vi "CreatePublicEvents.vi"(8 "error in (no error)":errorcluster, 11 "Generator":refnum<class "Generator.lvclass">) -> (0 "error out":errorcluster, 3 "Generator out":refnum<class "Generator.lvclass">)   [LabVIEW 2019, in "Generator.lvclass"]
uses:
  Generator.lvclass
  typedefs/AO.Channel--Cluster--Array.ctl
  typedefs/AO.Channel--Cluster.ctl
  typedefs/AO.Channel.Function--Enum.ctl
  typedefs/Waveforms--Cluster.ctl
  Generator.lvclass/Generator.ctl
  <vilib>/JKI/JKI SMO/SMO/SMO.lvclass
  typedefs/Generator.Sweep Status--enum.ctl
panel:
  # "For instructions on how to use the JKI State Machine Objects, examples and video tutorials, visit:\nhttp://jki.net/state-machine-objects/\n\nJKI State Machine Objects™\nhttp://jki.net/state-machine-objects/\nCopyright (C) 2005-2015, JKI <info@jki.net>\nALL RIGHTS RESERVED"
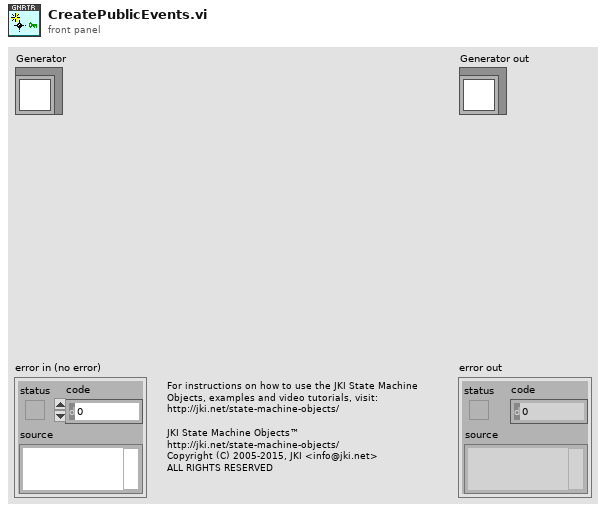
[diagram p1: front panel]
types:
  T1 = typedef "Generator.lvclass/Generator.Sweep Status--enum.ctl" = enum16{"idle", "initializing", "waiting", "sweeping", "stopping"}
  T2 = typedef "Generator.lvclass/Waveforms--Cluster.ctl" = cluster{"AO":waveform(dbl)[], "REF_X":waveform(dbl)[], "REF_Y":waveform(dbl)[]}
  T3 = typedef "Generator.lvclass/AO.Channel--Cluster--Array.ctl" = T4[]
  T4 = typedef "Generator.lvclass/AO.Channel--Cluster.ctl" = cluster{"Enable?":bool, "Channel":i32, "Amplitude":dbl, "Offset":dbl, "Frequency":dbl, "Phase":dbl, "Function":T5, "Sweeping?":bool, "Limit AC?":bool, "Limit DC?":bool, "Duty Cycle?":bool, "Duty Cycle":dbl}
  T5 = typedef "Generator.lvclass/AO.Channel.Function--Enum.ctl" = enum16{"sine", "square", "triangle", "saw"}
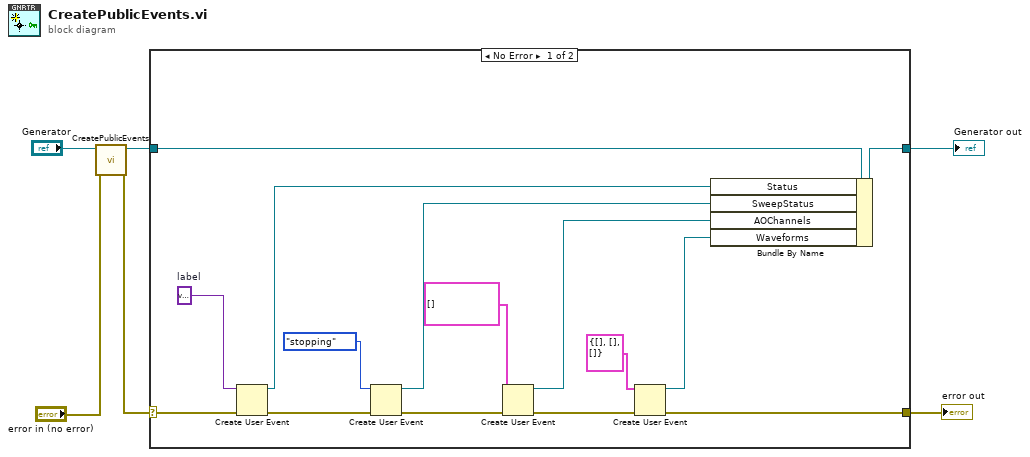
[diagram p0: block diagram]
diagram:
  n1 = call-parent "CreatePublicEvents.vi"("error in (no error)"="error in (no error)", "SMO"="Generator") -> ("error out"=w1:errorcluster, "SMO out"=w5:refnum<class "Generator.lvclass">)  [unwired: 8 in]
  n2 = case shown="No Error" w1 {
    selector: w1 -> [w20 w23]
    tunnel: [w12 w23] -> w3
    tunnel: [w21 w22] -> w4
    tunnel: w5 -> [w18 w22]
    frame No Error {
      w17 = variant  # label
      n3 = Create User Event(user event datatype=w17, error in=w20) -> (user event=w19:refnum<user-event>, error out=w16:errorcluster)
      n4 = Create User Event(user event datatype=Generator.Sweep_Status--enum."stopping" ("sweep status"), error in=w16) -> (user event=w15:refnum<user-event>, error out=w14:errorcluster)
      n5 = Create User Event(user event datatype=T3 [] ("AO Channels"), error in=w14) -> (user event=w8:refnum<user-event>, error out=w13:errorcluster)
      n6 = Create User Event(user event datatype=T2 {"AO"=[], "REF_X"=[], "REF_Y"=[]} ("Waveforms"), error in=w13) -> (user event=w9:refnum<user-event>, error out=w12:errorcluster)
      n7 = Bundle By Name(cluster=w18, "Status"=w19, "SweepStatus"=w15, "AOChannels"=w8, "Waveforms"=w9) -> (w21:refnum<class "Generator.lvclass">)
    }
    frame Error {
    }
  }
  "error out" <- w3
  "Generator out" <- w4
